vi "Get frame size.vi"(8 "error in (no error)":errorcluster, 11 "camera handle in":i16) -> (0 "error out":errorcluster, 1 "y size":u16, 2 "x size":u16, 3 "camera handle out":i16)   [LabVIEW 2012]
uses:
  Visual Studio/Cascade wrapper/Release/Cascade wrapper.dll
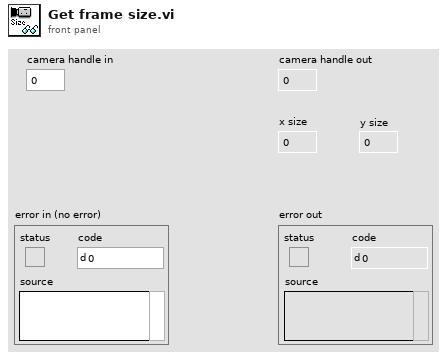
[diagram p1: front panel]
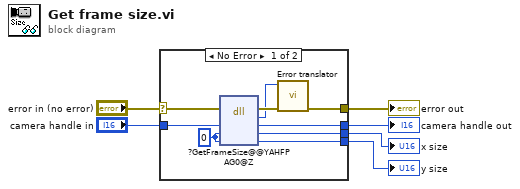
[diagram p0: block diagram]
diagram:
  n1 = case shown="No Error" "error in (no error)" {
    selector: "error in (no error)" -> [w15 w17]
    tunnel: "camera handle in" -> [w14 w16]
    tunnel: [w10 w17] -> w4
    tunnel: [w9 w16] -> w3
    tunnel: [w8 _] -> w2
    tunnel: [w7 _] -> w1
    frame No Error {
      w13 = u16 0 ("x size")
      n2 = dll-call lib="C:/moroder/Cascade wrapper/Visual Studio/Cascade wrapper/Release/Cascade wrapper.dll" fn="?GetFrameSize@@YAHFPAG0@Z"(error in=w15, "camera handle"=w14, "x size"=w13, "y size"=w13) -> (error out=w12:errorcluster, "error"=w11:i32, "camera handle"=w9:i16, "x size"=w8:u16, "y size"=w7:u16)  [unwired: 2 in, 1 out]
      n3 = call "Error translator.vi"("error in (no error)"=w12, "error code"=w11) -> ("error out"=w10:errorcluster)  [unwired: 9 in]
    }
    frame Error {
    }
  }
  "error out" <- w4
  "camera handle out" <- w3
  "x size" <- w2
  "y size" <- w1
